vi "GetPrice.vi"(8 "error in (no error)":errorcluster, 11 "Furniture in":refnum<class "Furniture.lvclass">) -> (0 "error out":errorcluster, 2 "Price":dbl, 3 "Furniture out":refnum<class "Furniture.lvclass">)   [LabVIEW 2019, in "Furniture.lvclass"]
uses:
  Furniture.lvclass
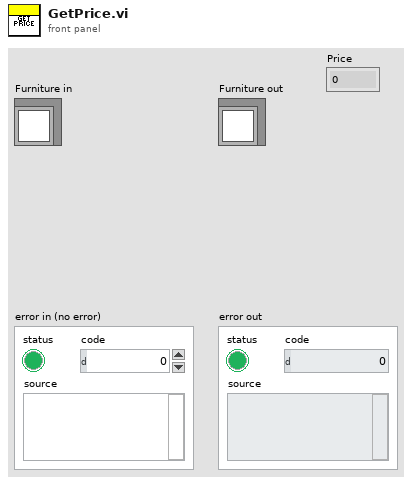
[diagram p1: front panel]
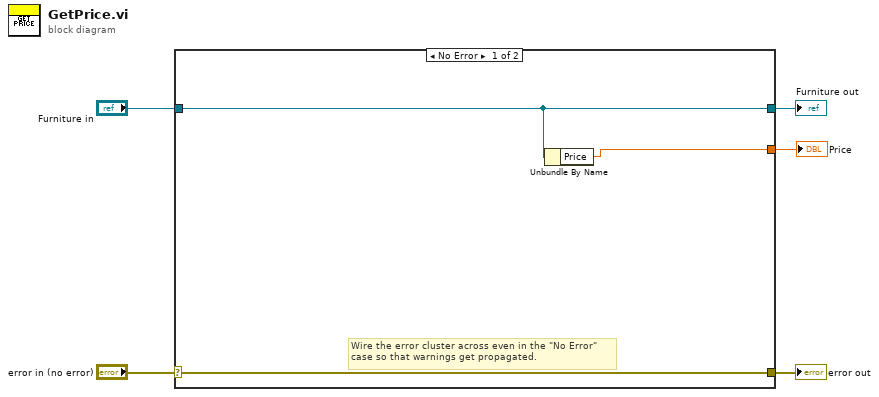
[diagram p0: block diagram]
diagram:
  n1 = case shown="No Error" "error in (no error)" {
    selector: "error in (no error)" -> [w8 w10]
    tunnel: [w8 w10] -> w2
    tunnel: [w7 w9] -> w4
    tunnel: "Furniture in" -> [w7 w9]
    tunnel: [w6 _] -> w1
    frame No Error {
      # "Wire the error cluster across even in the \"No Error\"\ncase so that warnings get propagated."
      n2 = Unbundle By Name(w7) -> ("Price"=w6:dbl)
    }
    frame Error {
    }
  }
  "Furniture out" <- w4
  "error out" <- w2
  "Price" <- w1
